vi "PhoroResistComparison.vi"() -> ()   [LabVIEW 2019]
uses:
  <vilib>/LabVIEW Interface for Arduino/Type Defs/Board Type.ctl
  <vilib>/LabVIEW Interface for Arduino/LabVIEW Interface for Arduino.lvlib
panel:
  out "Waveform Chart 2":dbl(graph)
  out "Intesity":dbl
  in  "stop":bool
  out "u":dbl
  out "Waveform Chart":dbl(graph)
  in  "Pin 1":u8
  out "error out":errorcluster
  in  "VISA resource":refnum<visa-resource-name>
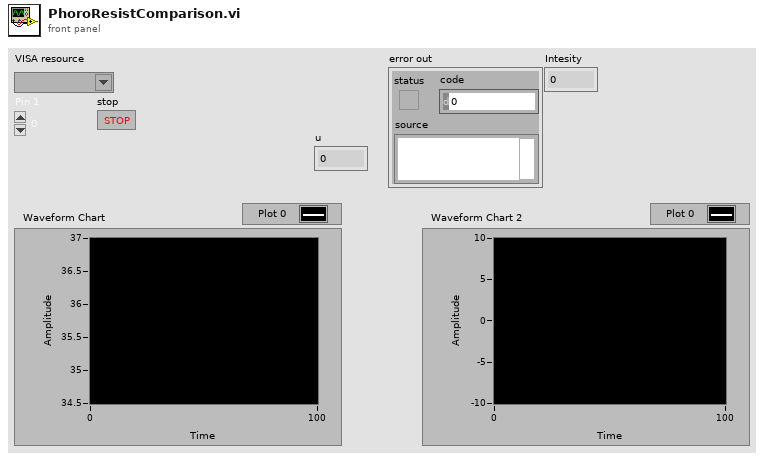
[diagram p1: front panel]
types:
  T1 = typedef "LabVIEW Interface for Arduino.lvlib/Board Type.ctl" = enum16{"Uno", "Dimuelanove w/Atmega 328", "Mega 2560"}
  T2 = typedef "LabVIEW Interface for Arduino.lvlib/Arduino Resource.ctl" = cluster{"VISA resource":refnum<visa-resource-name>, "Board Type":T1, "Connection Type":enum8{"USB / Serial"}, "Bytes Per Packet (15)":u8}
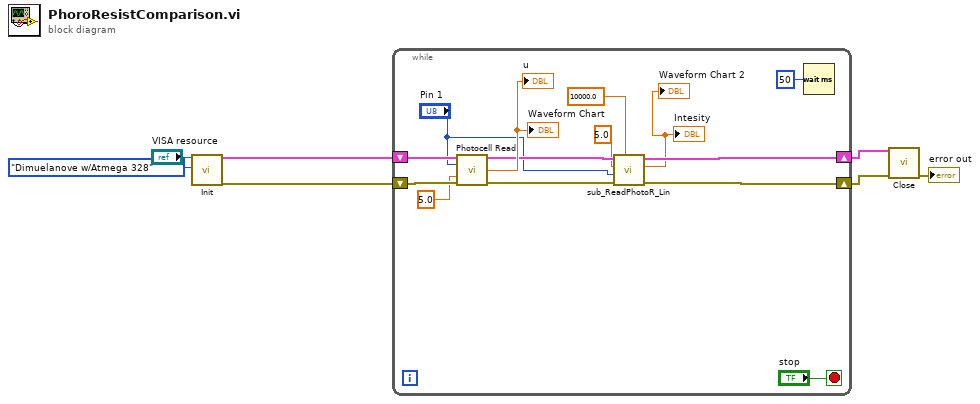
[diagram p0: block diagram]
diagram:
  n1 = call <vilib>:"Init.vi"("VISA resource"="VISA resource", "Board Type (Uno)"=Board_Type."Dimuelanove w/Atmega 328") -> ("Arduino Resource"=w5:T2, "error out"=w4:errorcluster)  [unwired: 16 in]
  n2 = while {
    shift-right: [w13] -> w3
    shift-left: w5 -> [w21]
    shift-right: [w12] -> w2
    shift-left: w4 -> [w20]
    stop <- "stop" stop-if-true
    n3 = call <vilib>:"Photocell Read.vi"("Arduino Resource"=w21, "Photo Cell Pin (0)"="Pin 1", "Vcc (5)"=5.0, "error in"=w20) -> ("Arduino Resource"=w15:T2, "Light Intensity (0 - 100)"=→"Waveform Chart" →"u":dbl, "error out"=w14:errorcluster)  [unwired: 9 in]
    n4 = call "sub_ReadPhotoR_Lin.vi"("Paired R (10kO)"=10000.0, "error in"=w14, "Analog Input Pin (0)"="Pin 1", "vcc (5V)"=5.0, "Arduino Resource"=w15) -> ("error out"=w12:errorcluster, "Intesity"=→"Intesity" →"Waveform Chart 2":dbl, "Arduino Resource 2"=w13:T2)  [unwired: 4 in]
    n5 = Wait (ms)(milliseconds to wait=u32 50) -> ()  [unwired: 1 out]
  }
  n6 = call <vilib>:"Close.vi"("Arduino Resource"=w3, "error in"=w2) -> ("error out"=→"error out":errorcluster)  [unwired: 13 in]
